vi "InitDialog.vi"(8 "error in (no error)":errorcluster, 10 "RT_Game.lvlib:Game.lvclass":refnum<class "Game.lvclass">, 11 "Highscore in":refnum<class "Highscore.lvclass">) -> (0 "error out":errorcluster, 2 "RT_Game.lvlib:Game.lvclass 2":refnum<class "Game.lvclass">, 3 "Highscore out":refnum<class "Highscore.lvclass">)   [LabVIEW 2019, in "RT_Game.lvlib" / "Highscore.lvclass"]
uses:
  Highscore.lvclass
  Game/Game.lvclass
  Engine/Coordinate.ctl
  Highscore.lvclass/Highscore.ctl
  Game/Game.lvclass/Game.ctl
  HighscoreDialog/HighscoreDialog.lvclass/HighscoreDialog.ctl
  GameObject/GameObject.lvclass/GameObject.ctl
  HighscoreDialog/Write Entries.vi
  HighscoreDialog/Write IndexInList.vi
  GameObject/Write IsActive.vi
  HighscoreDialog/Write IsLeft_.vi
  GameObject/Write position.vi
  Game/Read Player1Score.vi
  Game/Read Player2Score.vi
  Game/Read Singleplayer.vi
  HighscoreDialog/HighscoreDialog.lvclass
  C:/Users/FreshBob/Dropbox/VIs/myRIO_GameConsole/RT/RT_Game/GameObject/GameObject.lvclass
  Engine/Engine.lvclass
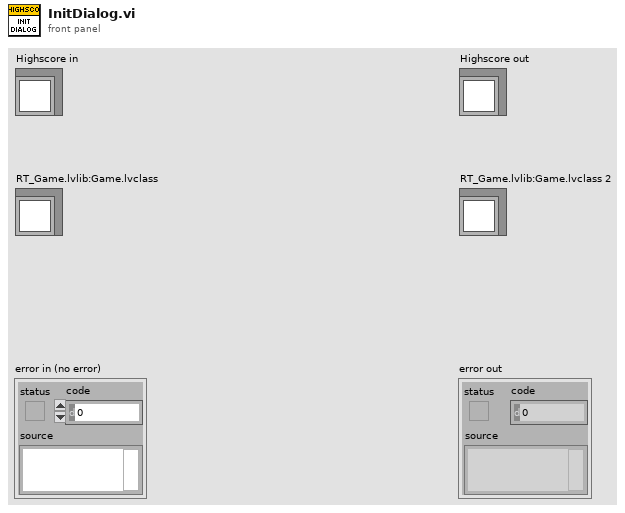
[diagram p1: front panel]
types:
  T1 = typedef "RT_Game.lvlib/Engine.lvclass/Coordinate.ctl" = cluster{"x":dbl, "y":dbl}
  T2 = typedef "RT_Game.lvlib/Highscore.lvclass/HighscoreEntry.ctl" = cluster{"Name":string, "Score":dbl}
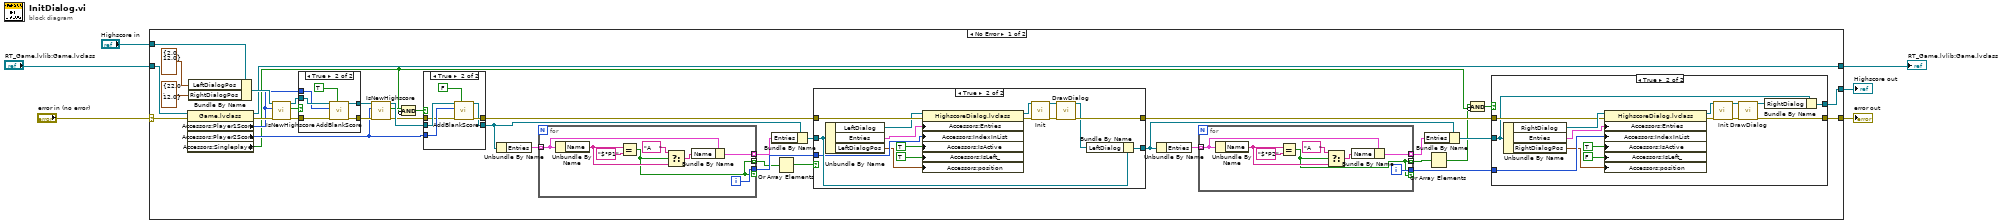
[diagram p0: block diagram]
diagram:
  n1 = case shown="No Error" "error in (no error)" {
    selector: "error in (no error)" -> [w45 w114]
    tunnel: [w25 w114] -> w5
    tunnel: [w24 w113] -> w3
    tunnel: "Highscore in" -> [w43 w113]
    tunnel: [w19 w112] -> w2
    tunnel: "RT_Game.lvlib:Game.lvclass" -> [w44 w112]
    frame No Error {
      n2 = property class="Game.lvclass"(reference=w44, error in=w45) -> (reference out=w19:refnum<class "Game.lvclass">, error out=w39:errorcluster, "Accessors:Player1Score"=w38:i32, "Accessors:Player2Score"=w30:i32, "Accessors:Singleplayer"=w17:bool)
      n3 = Bundle By Name(cluster=w43, "LeftDialogPos"=T1 {"x"=2.0, "y"=12.0}, "RightDialogPos"=T1 {"x"=22.0, "y"=12.0}) -> (w40:refnum<class "Highscore.lvclass">)
      n4 = call "IsNewHighscore.vi"("error in (no error)"=w39, "Score"=w38, "Highscore in"=w40) -> ("error out"=w37:errorcluster, "IsNewHighscore?"=w21:bool, "Highscore out"=w36:refnum<class "Highscore.lvclass">)  [unwired: 6 in]
      n5 = case shown="True" w21 {
        tunnel: w36 -> [w104 w111]
        tunnel: w38 -> [_ w110]
        tunnel: [w104 w107] -> w33
        tunnel: w37 -> [w105 w109]
        tunnel: [w105 w108] -> w32
        frame False {
        }
        frame True {
          n6 = call "AddBlankScore.vi"("P1?"=TRUE, "error in (no error)"=w109, "Accessors:Player1Score"=w110, "Highscore in"=w111) -> ("error out"=w108:errorcluster, "Highscore out"=w107:refnum<class "Highscore.lvclass">)  [unwired: 6 in]
        }
      }
      n7 = call "IsNewHighscore.vi"("error in (no error)"=w32, "Score"=w30, "Highscore in"=w33) -> ("error out"=w34:errorcluster, "IsNewHighscore?"=w22:bool, "Highscore out"=w35:refnum<class "Highscore.lvclass">)  [unwired: 6 in]
      n8 = Compound Arithmetic op=AND(w22, invert w17) -> (w20:bool)
      n9 = case shown="True" w20 {
        tunnel: w35 -> [w96 w103]
        tunnel: w30 -> [_ w102]
        tunnel: [w96 w98] -> w29
        tunnel: w34 -> [w97 w101]
        tunnel: [w97 w100] -> w31
        frame False {
        }
        frame True {
          n10 = call "AddBlankScore.vi"("P1?"=FALSE, "error in (no error)"=w101, "Accessors:Player1Score"=w102, "Highscore in"=w103) -> ("error out"=w100:errorcluster, "Highscore out"=w98:refnum<class "Highscore.lvclass">)  [unwired: 6 in]
        }
      }
      n11 = Unbundle By Name(w29) -> ("Entries"=w28:T2[])
      n12 = for {
        tunnel: w28 -> [w93] mode=indexing
        tunnel: [w94] -> w27 if=w88
        tunnel: [w88] -> w23 mode=indexing
        tunnel: [w92] -> w14 mode=indexing
        i -> [w94]
        n13 = Unbundle By Name(w93) -> ("Name"=w90:string)
        n14 = Equal?(x=w90, y="$°P1") -> (x = y?=w88:bool)
        n15 = Select(t="A    ", s=w88, f=w90) -> (s? t:f=w91:string)
        n16 = Bundle By Name(cluster=w93, "Name"=w91) -> (w92:T2)
      }
      n17 = Bundle By Name(cluster=w29, "Entries"=w14) -> (w15:refnum<class "Highscore.lvclass">)
      n18 = Or Array Elements(Boolean array=w23) -> (logical OR=w16:bool)
      n19 = case shown="True" w16 {
        tunnel: w31 -> [w71 w87]
        tunnel: w15 -> [w72 w84]
        tunnel: w27 -> [_ w83]
        tunnel: [w71 w77] -> w26
        tunnel: [w72 w81] -> w10
        frame False {
        }
        frame True {
          n20 = Unbundle By Name(w84) -> ("LeftDialog"=w86:refnum<class "HighscoreDialog.lvclass">, "Entries"=w85:T2[], "LeftDialogPos"=w73:T1)
          n21 = property class="HighscoreDialog.lvclass"(reference=w86, error in=w87, "Accessors:Entries"=w85, "Accessors:IndexInList"=w83, "Accessors:IsActive"=TRUE ("IsActive"), "Accessors:IsLeft_"=TRUE ("IsLeft_"), "Accessors:position"=w73) -> (reference out=w78:refnum<class "HighscoreDialog.lvclass">, error out=w82:errorcluster)
          n22 = call-dynamic "Init.vi"("error in (no error)"=w82, "HighscoreDialog in"=w78) -> ("error out"=w79:errorcluster, "HighscoreDialog out"=w76:refnum<class "HighscoreDialog.lvclass">)  [unwired: 8 in]
          n23 = call "DrawDialog.vi"("error in (no error)"=w79, "Highscore in"=w76) -> ("error out"=w77:errorcluster, "Highscore out"=w75:refnum<class "HighscoreDialog.lvclass">)  [unwired: 8 in]
          n24 = Bundle By Name(cluster=w84, "LeftDialog"=w75) -> (w81:refnum<class "Highscore.lvclass">)
        }
      }
      n25 = Unbundle By Name(w10) -> ("Entries"=w11:T2[])
      n26 = for {
        tunnel: w11 -> [w51] mode=indexing
        tunnel: [w52] -> w7 if=w46
        tunnel: [w46] -> w12 mode=indexing
        tunnel: [w50] -> w13 mode=indexing
        i -> [w52]
        n27 = Unbundle By Name(w51) -> ("Name"=w48:string)
        n28 = Equal?(x=w48, y="$°P2") -> (x = y?=w46:bool)
        n29 = Select(t="A    ", s=w46, f=w48) -> (s? t:f=w49:string)
        n30 = Bundle By Name(cluster=w51, "Name"=w49) -> (w50:T2)
      }
      n31 = Bundle By Name(cluster=w10, "Entries"=w13) -> (w9:refnum<class "Highscore.lvclass">)
      n32 = Or Array Elements(Boolean array=w12) -> (logical OR=w8:bool)
      n33 = Compound Arithmetic op=AND(w8, invert w17) -> (w18:bool)
      n34 = case shown="True" w18 {
        tunnel: w7 -> [_ w70]
        tunnel: w26 -> [w54 w67]
        tunnel: [w54 w60] -> w25
        tunnel: w9 -> [w55 w65]
        tunnel: [w55 w64] -> w24
        frame False {
        }
        frame True {
          n35 = Unbundle By Name(w65) -> ("RightDialog"=w68:refnum<class "HighscoreDialog.lvclass">, "Entries"=w69:T2[], "RightDialogPos"=w56:T1)
          n36 = property class="HighscoreDialog.lvclass"(reference=w68, error in=w67, "Accessors:Entries"=w69, "Accessors:IndexInList"=w70, "Accessors:IsActive"=TRUE ("IsActive"), "Accessors:IsLeft_"=FALSE ("IsLeft_"), "Accessors:position"=w56) -> (reference out=w61:refnum<class "HighscoreDialog.lvclass">, error out=w66:errorcluster)
          n37 = call-dynamic "Init.vi"("error in (no error)"=w66, "HighscoreDialog in"=w61) -> ("error out"=w62:errorcluster, "HighscoreDialog out"=w59:refnum<class "HighscoreDialog.lvclass">)  [unwired: 8 in]
          n38 = call "DrawDialog.vi"("error in (no error)"=w62, "Highscore in"=w59) -> ("error out"=w60:errorcluster, "Highscore out"=w58:refnum<class "HighscoreDialog.lvclass">)  [unwired: 8 in]
          n39 = Bundle By Name(cluster=w65, "RightDialog"=w58) -> (w64:refnum<class "Highscore.lvclass">)
        }
      }
    }
    frame Error {
    }
  }
  "error out" <- w5
  "Highscore out" <- w3
  "RT_Game.lvlib:Game.lvclass 2" <- w2
